vi "IMAQ LL-Snap.vi"(7 "ImgName":string="untitled", 8 "ErrIn":errorcluster, 11 "IF Name":string="img0") -> (0 "ErrOut":errorcluster, 3 "ImgOut":T1)   [LabVIEW 2013]
doc: "Use this template to build a VI to use as a subVI."
uses:
  <vilib>/vision/Image Controls.llb/IMAQ Image.ctl
panel:
  # "Input Parameters"
  # "Output Parameters"
  # "VI Description:\nThis VI is created to snap a image from imaging device."
  # ":: MVI Framework V1.0 ::\nAuthor:Gaoke Yang\nEmail: gaoke.yang@yahoo.com\nWeb: www.mvicontrol.com\nCopyright (C) 2013, MVI Technologies All Rights Reserved"
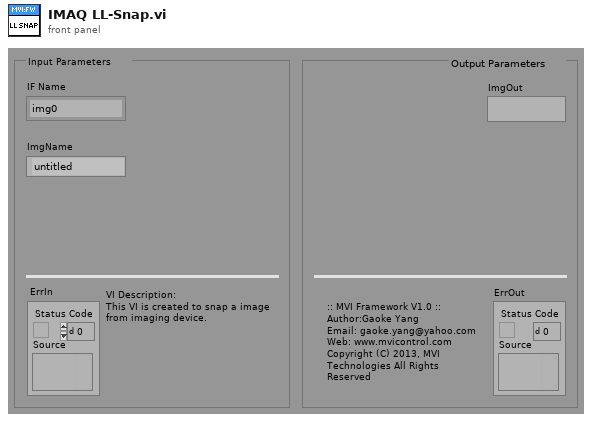
[diagram p1: front panel]
types:
  T1 = typedef "IMAQ Image.ctl" = refnum<image>
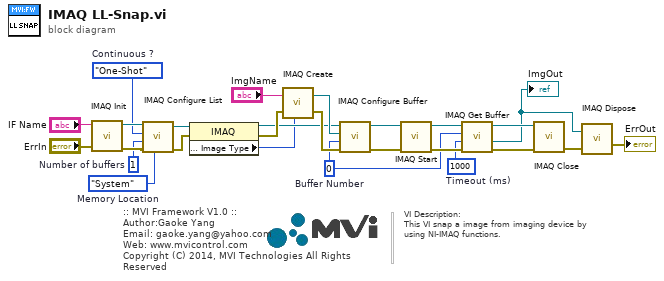
[diagram p0: block diagram]
diagram:
  w16 = 1000  # Timeout (ms)
  w17 = enum16{"System", "Onboard"}."System"  # Memory Location
  w1 = u32 0  # Buffer Number
  w2 = u32 1  # Number of buffers
  w25 = enum16{"One-Shot", "Continuous"}."One-Shot"  # Continuous ?
  # "VI Description:\nThis VI snap a image from imaging device by\nusing NI-IMAQ functions."
  # ":: MVI Framework V1.0 ::\nAuthor:Gaoke Yang\nEmail: gaoke.yang@yahoo.com\nWeb: www.mvicontrol.com\nCopyright (C) 2014, MVI Technologies All Rights Reserved"
  n1 = call <vilib>:"IMAQ Init.vi"("error in (no error)"="ErrIn", "Interface Name"="IF Name") -> ("error out"=w24:errorcluster, "IMAQ Session Out"=w26:refnum<k11>)  [unwired: 8 out]
  n2 = call <vilib>:"IMAQ Configure List.vi"("Memory Location"=w17, "error in (no error)"=w24, "Number of buffers"=w2, "Continuous?"=w25, "IMAQ Session In"=w26) -> ("error out"=w14:errorcluster, "IMAQ Session Out"=w15:refnum<k11>)  [unwired: 1 in, 4 out]
  n3 = property class="IMAQ"(reference=w15, error in=w14) -> (reference out=w12:refnum<k11>, error out=w13:errorcluster, "Image Parameters : Image Type"=w11:u32)
  n4 = call "IMAQ Create"("Image Name"="ImgName", "Image Type"=w11, "error in (no error)"=w13) -> ("New Image"=w22:T1, "error out"=w23:errorcluster)  [unwired: 1 in, 1 out]
  n5 = call <vilib>:"IMAQ Configure Buffer.vi"("error in (no error)"=w23, "Buffer Number"=w1, "Image In"=w22, "IMAQ Session In"=w12) -> ("error out"=w21:errorcluster, "IMAQ Session Out"=w20:refnum<k11>)  [unwired: 2 in, 4 out]
  n6 = call <vilib>:"IMAQ Start.vi"("error in (no error)"=w21, "IMAQ Session In"=w20) -> ("error out"=w19:errorcluster, "IMAQ Session Out"=w18:refnum<k11>)  [unwired: 8 out]
  n7 = call <vilib>:"IMAQ Get Buffer.vi"("error in (no error)"=w19, "Timeout (ms)"=w16, "Buffer Number (-1:all)"=w1, "IMAQ Session In"=w18) -> ("error out"=w5:errorcluster, "Image Out"=w4:T1, "IMAQ Session Out"=w6:refnum<k11>)  [unwired: 5 out]
  "ImgOut" <- w4
  n8 = call <vilib>:"IMAQ Close.vi"("error in (no error)"=w5, "IMAQ Session In"=w6) -> ("error out"=w10:errorcluster)  [unwired: 9 out]
  n9 = call "IMAQ Dispose"("Image"=w4, "error in (no error)"=w10) -> ("error out"=→"ErrOut":errorcluster)  [unwired: 1 in, 3 out]
